vi "Convert Assert Event Data to Test Case - Time is Zero - Time is calculated from Timestamp.vi"() -> ()   [LabVIEW 2013, in "JUnit Conversion Tests.lvlib"]
uses:
  JUnit Conversion Tests.lvlib
  JUnit Conversion/JUnit Conversion.lvlib
  <vilib>/addons/_JKI Toolkits/Caraya/classes/Test Result/Assert Event Data (Extended).ctl
  <vilib>/addons/_JKI Toolkits/Caraya/classes/Test Result/Test Result.lvclass
  <vilib>/addons/_JKI Toolkits/Caraya/classes/Assert/Assert.lvclass
  <vilib>/addons/_JKI Toolkits/Caraya/classes/Assert/Assert Equal Value_Variant.vi
  <vilib>/addons/_JKI Toolkits/Caraya/classes/Test/Test.lvclass
  <vilib>/PNR/JUnit XML/JUnit XML/Test Case/Test Case.lvclass
panel:
  out "error out":errorcluster
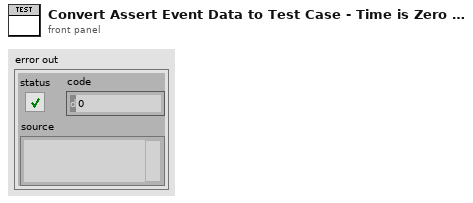
[diagram p1: front panel]
types:
  T1 = typedef "Caraya.lvlib/Test Result.lvclass/Assert Event Data (Extended).ctl" = cluster{"name":string, "passed":bool, "call-chain":string[], "test-error":errorcluster, "timestamp":timestamp, "assert-id":string, "test-id":string, "time":dbl, "message":string, "properties":variant, "measurements":variant, "user-defined":variant}
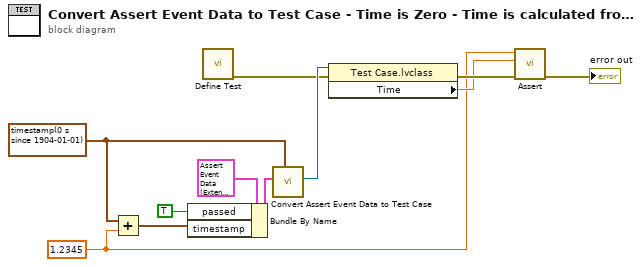
[diagram p0: block diagram]
diagram:
  w1 = 1.2345 ("time")
  w2 = timestamp(0 s since 1904-01-01) ("Start Time")
  n1 = Add(x=w2, y=w1) -> (x+y=w3:timestamp)
  n2 = Bundle By Name(cluster=T1 {"name"="", "passed"=FALSE, "call-chain"=[], "test-error"={"status"=FALSE, "code"=0, "source"=""}, "timestamp"=timestamp(0 s since 1904-01-01), "assert-id"="", "test-id"="", "time"=-1.0, "message"="", "properties"=variant, "measurements"=variant, "user-defined"=variant} ("Assert Event Data"), "passed"=TRUE, "timestamp"=w3) -> (w10:T1)
  n3 = call <vilib>:"Define Test.vi"() -> ("error out"=w5:errorcluster)  [unwired: 10 in, 1 out]
  n4 = call "Convert Assert Event Data to Test Case.vi"("Start Time"=w2, "Assert Event Data"=w10) -> ("Test Case"=w9:refnum<class "Test Case.lvclass">)  [unwired: 9 in]
  n5 = property class="Test Case.lvclass"(reference=w9, error in=w5) -> (error out=w7:errorcluster, "Time"=w6:dbl)  [unwired: 1 out]
  n6 = call-poly <vilib>:"Assert.vi"("error in (no error)"=w7, "Actual"=w6, "Expected"=w1) -> ("error out"=→"error out":errorcluster)  [unwired: 7 in, 1 out]
